vi "CAN RESPONSE.vi"() -> ()   [LabVIEW 2017]
uses:
  <vilib>/Utility/file.llb/Write Delimited Spreadsheet (string).vi
  <vilib>/Utility/file.llb/Read Delimited Spreadsheet (string).vi
panel:
  out "all rows":string[][](array[string])
  out "error out 2":errorcluster
  in  "array w/ subset deleted 3":string[][](array[string])
  out "array w/ subset deleted 2":string[][](array[string])
  out "error out":errorcluster
  out "Array":string[][](array[string])
  in  "CAN Table":string[][](table)=[["time", "301", "CAN Data Frame", "3", "59 E2 53 0 0 0 0 0", ""], ["time", "301", "CAN Data Frame", "3", "59 E2 52 0 0 0 0 0", ""], ["time", "301", "CAN Data Frame", "3", "59 E2 52 0 0 0 0 0", ""], ["time", "301", "CAN Data Frame", "3", "59 E2 52 0 0 0 0 0", ""], ["11:04:17.477", "20000302", "CAN Data Frame\r\n", " 4", "99\tEE\t51\t00\r\n", ""], ["time", "301", "CAN Data Frame", "3", "59 E2 51 0 0 0 0 0", ""], ["10:59:00.638", "20000302", "CAN Data Frame\r\n", " 7", "99\t65\t02\t32\t37\t37\t37\r\n", ""], ["10:59:00.638", "20000302", "CAN Data Frame\r\n", " 7", "99\t65\t01\t31\t44\t30\t30\r\n", ""], ["time", "301", "CAN Data Frame", "3", "59 E2 65 0 0 0 0 0", ""], ["10:58:21.536", "20000302", "CAN Data Frame\r\n", " 8", "99\t63\tFF\tFF\tFF\tFF\tFF\tFF\r\n", ""], ["time", "301", "CAN Data Frame", "3", "59 E2 63 0 0 0 0 0", ""], ["10:55:02.505", "20000302", "CAN Data Frame\r\n", " 7", "99\t66\t01\t50\t4D\t50\t33\r\n", ""], ["time", "301", "CAN Data Frame", "3", "59 E2 66 0 0 0 0 0", ""], ["10:47:02.016", "20000302", "CAN Data Frame\r\n", " 5", "99\tEE\t10\t0C\tDE\r\n", ""], ["time", "301", "CAN Data Frame", "3", "59 E3 10 0 0 0 0 0", ""], ["10:46:44.511", "20000302", "CAN Data Frame\r\n", " 4", "99\tEE\t25\t01\r\n", ""], ["time", "301", "CAN Data Frame", "3", "59 E3 25 0 0 0 0 0", ""], ["10:46:41.912", "20000302", "CAN Data Frame\r\n", " 4", "99\tEE\t24\t00\r\n", ""], ["time", "301", "CAN Data Frame", "3", "59 E3 24 0 0 0 0 0", ""], ["10:46:39.613", "20000302", "CAN Data Frame\r\n", " 4", "99\tEE\t23\t00\r\n", ""], ["time", "301", "CAN Data Frame", "3", "59 E3 23 0 0 0 0 0", ""], ["10:46:37.113", "20000302", "CAN Data Frame\r\n", " 4", "99\tEE\t22\t01\r\n", ""], ["time", "301", "CAN Data Frame", "3", "59 E3 22 0 0 0 0 0", ""], ["10:46:34.410", "20000302", "CAN Data Frame\r\n", " 4", "99\tEE\t21\t00\r\n", ""], ["time", "301", "CAN Data Frame", "3", "59 E3 21 0 0 0 0 0", ""], ["10:46:20.110", "20000302", "CAN Data Frame\r\n", " 4", "99\tEE\t20\t00\r\n", ""], ["time", "301", "CAN Data Frame", "3", "59 E3 20 0 0 0 0 0", ""], ["10:46:14.210", "20000302", "CAN Data Frame\r\n", " 4", "99\tEE\t76\t00\r\n", ""], ["time", "301", "CAN Data Frame", "3", "59 E4 76 0 0 0 0 0", ""], ["10:46:11.109", "20000302", "CAN Data Frame\r\n", " 4", "99\tEE\t75\t00\r\n", ""], ["time", "301", "CAN Data Frame", "3", "59 E4 75 0 0 0 0 0", ""], ["10:46:08.510", "20000302", "CAN Data Frame\r\n", " 4", "99\tEE\t74\t00\r\n", ""], ["time", "301", "CAN Data Frame", "3", "59 E4 74 0 0 0 0 0", ""], ["10:46:03.607", "20000302", "CAN Data Frame\r\n", " 4", "99\tEE\t73\t00\r\n", ""], ["time", "301", "CAN Data Frame", "3", "59 E4 73 0 0 0 0 0", ""], ["10:45:33.103", "20000302", "CAN Data Frame\r\n", " 4", "99\tEE\t72\t00\r\n", ""], ["time", "301", "CAN Data Frame", "3", "59 E4 72 0 0 0 0 0", ""], ["10:45:20.602", "20000302", "CAN Data Frame\r\n", " 4", "99\tEE\t71\t00\r\n", ""], ["time", "301", "CAN Data Frame", "3", "59 E4 71 0 0 0 0 0", ""], ["10:45:14.602", "20000302", "CAN Data Frame\r\n", " 4", "99\tEE\t86\t01\r\n", ""], ["time", "301", "CAN Data Frame", "3", "59 E4 86 0 0 0 0 0", ""], ["10:45:11.501", "20000302", "CAN Data Frame\r\n", " 4", "99\tEE\t85\t01\r\n", ""], ["time", "301", "CAN Data Frame", "3", "59 E4 85 0 0 0 0 0", ""], ["10:45:08.301", "20000302", "CAN Data Frame\r\n", " 4", "99\tEE\t84\t01\r\n", ""], ["time", "301", "CAN Data Frame", "3", "59 E4 84 0 0 0 0 0", ""], ["10:45:03.699", "20000302", "CAN Data Frame\r\n", " 4", "99\tEE\t83\t01\r\n", ""], ["time", "301", "CAN Data Frame", "3", "59 E4 83 0 0 0 0 0", ""], ["10:44:59.897", "20000302", "CAN Data Frame\r\n", " 4", "99\tEE\t82\t01\r\n", ""], ["time", "301", "CAN Data Frame", "3", "59 E4 82 0 0 0 0 0", ""], ["10:44:53.797", "20000302", "CAN Data Frame\r\n", " 4", "99\tEE\t81\t01\r\n", ""], ["time", "301", "CAN Data Frame", "3", "59 E4 81 0 0 0 0 0", ""], ["10:44:29.395", "20000302", "CAN Data Frame\r\n", " 4", "7F\t59\t86\t13\r\n", ""], ["time", "301", "CAN Data Frame", "3", "59 E2 86 0 0 0 0 0", ""], ["10:44:22.293", "20000302", "CAN Data Frame\r\n", " 4", "7F\t59\t85\t13\r\n", ""], ["time", "301", "CAN Data Frame", "3", "59 E2 85 0 0 0 0 0", ""], ["10:44:16.794", "20000302", "CAN Data Frame\r\n", " 4", "7F\t59\t84\t13\r\n", ""], ["time", "301", "CAN Data Frame", "3", "59 E2 84 0 0 0 0 0", ""], ["10:44:10.794", "20000302", "CAN Data Frame\r\n", " 4", "7F\t59\t83\t13\r\n", ""], ["time", "301", "CAN Data Frame", "3", "59 E2 83 0 0 0 0 0", ""], ["10:44:04.393", "20000302", "CAN Data Frame\r\n", " 4", "7F\t59\t82\t13\r\n", ""], ["time", "301", "CAN Data Frame", "3", "59 E2 82 0 0 0 0 0", ""], ["10:43:27.285", "20000302", "CAN Data Frame\r\n", " 4", "7F\t59\t81\t13\r\n", ""], ["time", "301", "CAN Data Frame", "3", "59 E2 81 0 0 0 0 0", ""], ["10:43:01.983", "20000302", "CAN Data Frame\r\n", " 7", "99\t64\t40\t01\t40\t14\t40\r\n", ""], ["time", "301", "CAN Data Frame", "3", "59 E2 64 0 0 0 0 0", ""], ["10:39:18.160", "20000302", "CAN Data Frame\r\n", " 8", "99\t63\tFF\tFF\tFF\tFF\tFF\tFF\r\n", ""], ["time", "301", "CAN Data Frame", "3", "59 E2 63 0 0 0 0 0", ""], ["10:37:45.853", "20000302", "CAN Data Frame\r\n", " 5", "99\tEE\t6A\t02\t10\r\n", ""], ["time", "301", "CAN Data Frame", "3", "59 E2 6A 0 0 0 0 0", ""], ["10:34:23.607", "20000302", "CAN Data Frame\r\n", " 5", "99\tEE\t69\t01\t13\r\n", ""], ["time", "301", "CAN Data Frame", "3", "59 E2 69 0 0 0 0 0", ""], ["10:34:08.594", "20000302", "CAN Data Frame\r\n", " 3", "99\t00\t00\r\n", ""], ["time", "301", "CAN Data Frame", "3", "59 2A 76 0 0 0 0 0", ""], ["time", "301", "CAN Data Frame", "3", "59 2A 76 0 0 0 0 0", ""], ["10:34:05.694", "20000302", "CAN Data Frame\r\n", " 3", "99\t12\t5A\r\n", ""], ["time", "301", "CAN Data Frame", "1", "59 2A 76 0 0 0 0 0", ""], ["10:33:58.792", "20000302", "CAN Data Frame\r\n", " 3", "99\t12\t5A\r\n", ""], ["", "", "", "", "", ""], ["", "", "", "", "", ""], ["", "", "", "", "", ""], ["", "", "", "", "", ""], ["", "", "", "", "", ""], ["", "", "", "", "", ""], ["", "", "", "", "", ""], ["", "", "", "", "", ""], ["", "", "", "", "", ""], ["", "", "", "", "", ""], ["", "", "", "", "", ""], ["", "", "", "", "", ""], ["", "", "", "", "", ""], ["", "", "", "", "", ""], ["", "", "", "", "", ""]]
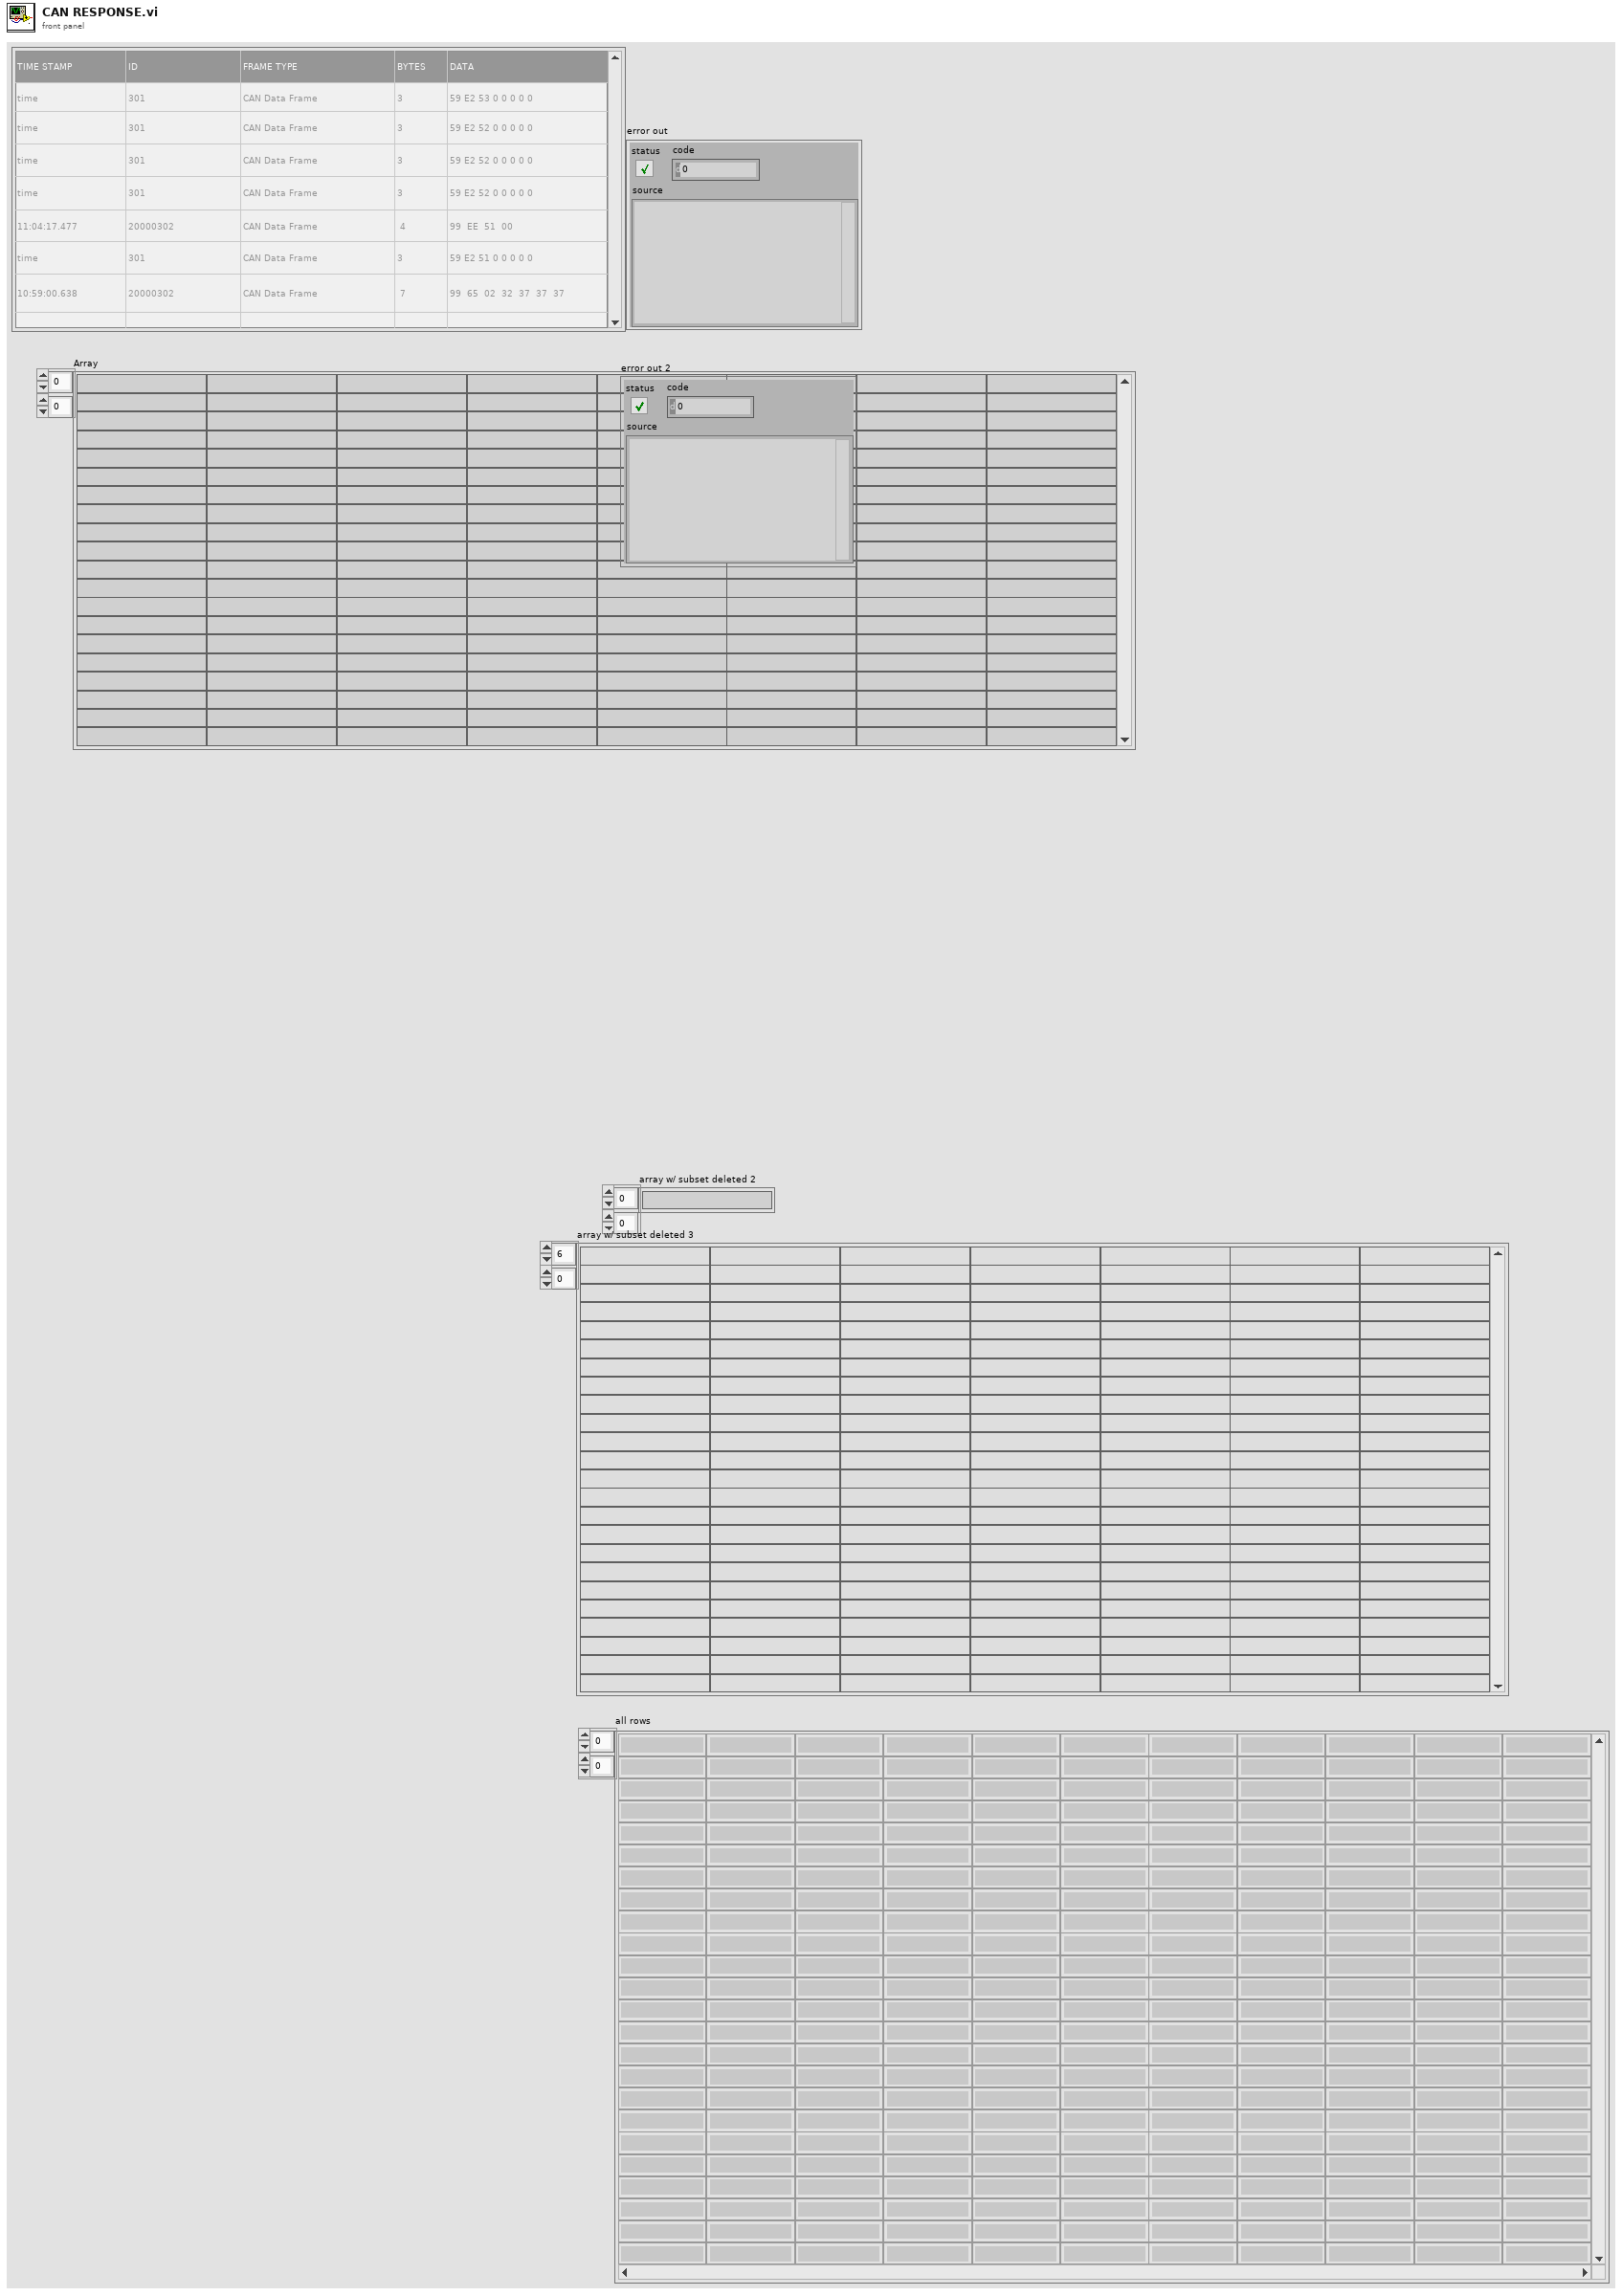
[diagram p1: front panel]
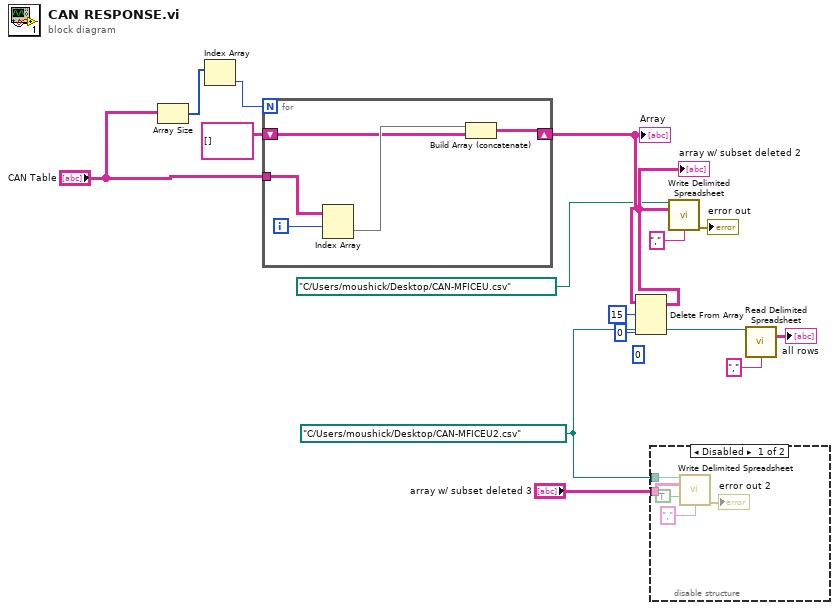
[diagram p0: block diagram]
diagram:
  w3 = path "C:/Users/moushick/Desktop/CAN-MFICEU2.csv" ("file path (dialog if empty)")
  (unwired) 0 ("index")
  n1 = Array Size(array="CAN Table") -> (size(s)=w13:i32[])
  n2 = Index Array(array=w13) -> (element=w12:i32)  [unwired: 1 in]
  n3 = for {
    N: w12 -> [_]
    tunnel: "CAN Table" -> [w19]
    shift-right: [w20] -> w9
    shift-left: string[][] [] -> [w16]
    i -> [w18]
    n4 = Index Array(array=w19, index (row)=w18) -> (element=w17:string[])  [unwired: 1 in]
    n5 = Build Array (concatenate)(w17, w16) -> (w20:string[][])
  }
  "Array" <- w9
  n6 = Delete From Array(array=w9, length=15, index (row)=0) -> (array with subset deleted=w6:string[][])  [unwired: 1 in, 1 out]
  "array w/ subset deleted 2" <- w6
  n7 = disable-structure shown="Disabled" {
    disable-tunnel: "array w/ subset deleted 3" -> [w23 _]
    disable-tunnel: w3 -> [w21 _]
    frame Disabled {
      n8 = call-poly <vilib>:"Write Delimited Spreadsheet.vi"("file path (dialog if empty)"=w21, "2D data"=w23, "append to file? (new file:F)"=TRUE, "delimiter (\\t)"="," ("delimiter (\\t)")) -> ("error out"=→"error out 2":errorcluster)  [unwired: 10 in, 1 out]
    }
    frame Enabled {
    }
  }
  n9 = call-poly <vilib>:"Write Delimited Spreadsheet.vi"("file path (dialog if empty)"=path "C:/Users/moushick/Desktop/CAN-MFICEU.csv", "2D data"=w6, "delimiter (\\t)"="," ("delimiter (\\t)")) -> ("error out"=→"error out":errorcluster)  [unwired: 11 in, 1 out]
  n10 = call-poly <vilib>:"Read Delimited Spreadsheet.vi"("file path (dialog if empty)"=w3, "delimiter (\\t)"="," ("delimiter (\\t)")) -> ("all rows"=→"all rows":string[][])  [unwired: 8 in, 5 out]
